vi "Strcat and Reverse.vi"(1 "stringB":string, 2 "stringA":string) -> (0 "CatAndReverse":string)   [LabVIEW 2012]
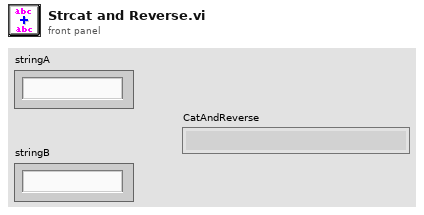
[diagram p1: front panel]
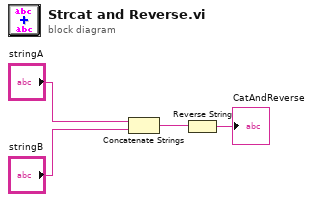
[diagram p0: block diagram]
diagram:
  n1 = Concatenate Strings("stringA", "stringB") -> (w2:string)
  n2 = Reverse String(1:w2) -> (0:→"CatAndReverse":string)
